vi "CRYGet Info From Channel Name.vi"(10 "Channel Name":string, 11 "Hardware In":string) -> (2 "In_ChannelInfo":T1={"ID"=0, "Name"="", "Digital"=FALSE, "Input"=FALSE, "Device Name"="", "Hardware Ch ID"=0, "Vmax (V)"=0.0, "Latency (samples)"=0.0, "Sampling Rate (Hz)"=0, "Bit Depth"=0, "Anti-aliasing Factor (%fs)"=0.0, "DAQmx Channel"="", "term config"=-1, "Coupling"=0, "IEPE en"=FALSE, "ASIOChannel Name"="", "Audio Driver"=0, "ASIOChannel Index"=0} {"Coupling" items=["Default"=-1, "RSE"=10083, "NRSE"=10078, "Differential"=10106, "Pseudodifferential"=12529]; "term config" items=["Default"=-1, "RSE"=10083, "NRSE"=10078, "Differential"=10106, "Pseudodifferential"=12529]; "Anti-aliasing Factor (%fs)" format="%.2f"}, 3 "Out_ChannelInfo":T1={"ID"=0, "Name"="", "Digital"=FALSE, "Input"=FALSE, "Device Name"="", "Hardware Ch ID"=0, "Vmax (V)"=0.0, "Latency (samples)"=0.0, "Sampling Rate (Hz)"=0, "Bit Depth"=0, "Anti-aliasing Factor (%fs)"=0.0, "DAQmx Channel"="", "term config"=-1, "Coupling"=0, "IEPE en"=FALSE, "ASIOChannel Name"="", "Audio Driver"=0, "ASIOChannel Index"=0} {"Coupling" items=["Default"=-1, "RSE"=10083, "NRSE"=10078, "Differential"=10106, "Pseudodifferential"=12529]; "term config" items=["Default"=-1, "RSE"=10083, "NRSE"=10078, "Differential"=10106, "Pseudodifferential"=12529]; "Anti-aliasing Factor (%fs)" format="%.2f"})   [LabVIEW 2013]
uses:
  Typedef Control/CRYHardware Channel Info.ctl
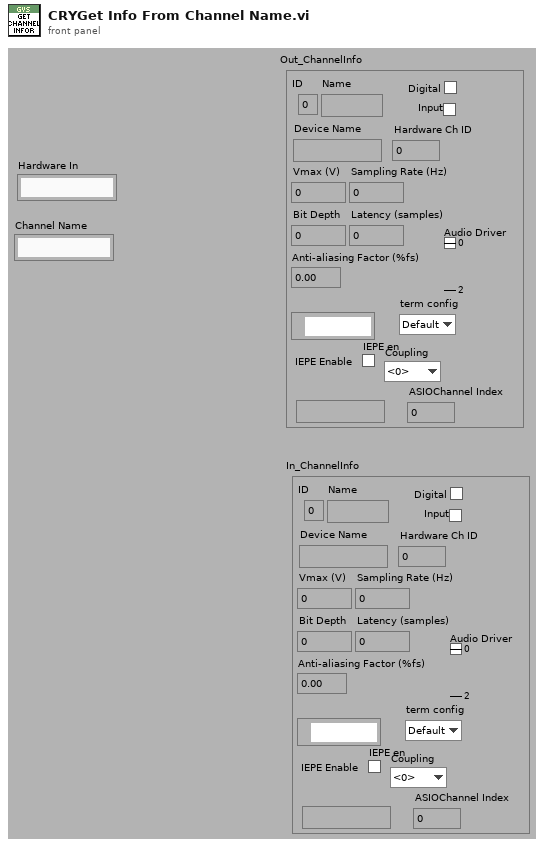
[diagram p1: front panel]
types:
  T1 = typedef "CRYHardware Channel Info.ctl" = cluster{"ID":i32, "Name":string, "Digital":bool, "Input":bool, "Device Name":string, "Hardware Ch ID":u8, "Vmax (V)":dbl, "Latency (samples)":dbl, "Sampling Rate (Hz)":u32, "Bit Depth":u32, "Anti-aliasing Factor (%fs)":sgl, "DAQmx Channel":tag, "term config":i32, "Coupling":i32, "IEPE en":bool, "ASIOChannel Name":string, "Audio Driver":u16, "ASIOChannel Index":u8}
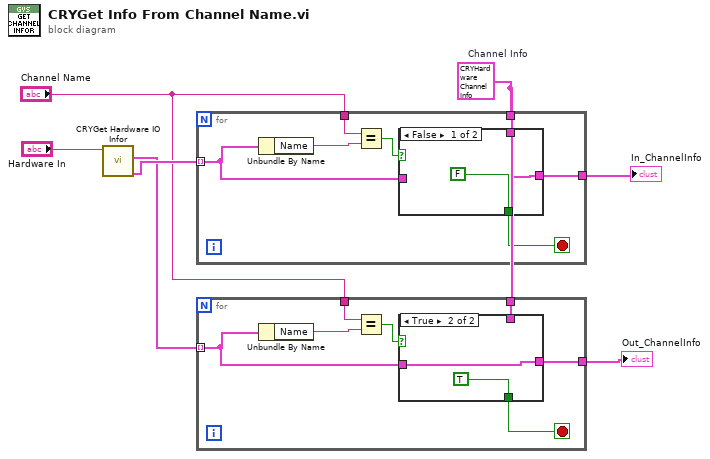
[diagram p0: block diagram]
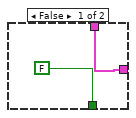
[diagram p2: hidden frame]
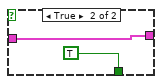
[diagram p3: hidden frame]
diagram:
  w2 = T1 {"ID"=0, "Name"="", "Digital"=FALSE, "Input"=FALSE, "Device Name"="", "Hardware Ch ID"=0, "Vmax (V)"=0.0, "Latency (samples)"=0.0, "Sampling Rate (Hz)"=0, "Bit Depth"=0, "Anti-aliasing Factor (%fs)"=0.475, "DAQmx Channel"="", "term config"=0, "Coupling"=-1, "IEPE en"=FALSE, "ASIOChannel Name"="", "Audio Driver"=0, "ASIOChannel Index"=0}  # Channel Info
  n1 = call "CRYGet Hardware IO Infor.vi"("Hardware setup In"="Hardware In") -> ("I_channel Info Out"=w6:T1[], "O_channel Info Out"=w4:T1[])  [unwired: 9 out]
  n2 = for {
    tunnel: w6 -> [w9] mode=indexing
    tunnel: [w13] -> w5
    tunnel: "Channel Name" -> [w12]
    tunnel: w2 -> [w8]
    stop <- w14 stop-if-true
    n3 = Unbundle By Name(w9) -> ("Name"=w11:string)
    n4 = Equal?(x=w12, y=w11) -> (x = y?=w10:bool)
    n5 = case shown="False" w10 {
      tunnel: [FALSE TRUE] -> w14
      tunnel: [w15 w17] -> w13
      tunnel: w9 -> [_ w17]
      tunnel: w8 -> [w15 _]
      frame False {
      }
      frame True {
      }
    }
  }
  "In_ChannelInfo" <- w5
  n6 = for {
    tunnel: w4 -> [w20] mode=indexing
    tunnel: [w24] -> w1
    tunnel: "Channel Name" -> [w23]
    tunnel: w2 -> [w19]
    stop <- w25 stop-if-true
    n7 = Unbundle By Name(w20) -> ("Name"=w22:string)
    n8 = Equal?(x=w23, y=w22) -> (x = y?=w21:bool)
    n9 = case shown="True" w21 {
      tunnel: [FALSE TRUE] -> w25
      tunnel: [w26 w28] -> w24
      tunnel: w20 -> [_ w28]
      tunnel: w19 -> [w26 _]
      frame False {
      }
      frame True {
      }
    }
  }
  "Out_ChannelInfo" <- w1
